vi "Stop Core.vi"(10 "final error code":i32, 11 "Debug UI in":refnum<class "Debug UI.lvclass">) -> (3 "Debug UI out":refnum<class "Debug UI.lvclass">)   [LabVIEW 2018, in "Assert API Components.lvlib" / "Log Assert Core.lvlib" / "Debug UI.lvclass"]
doc: "(<B>Filename</B>: Actor Framework.lvlib:Actor.lvclass:Stop Core.vi)\n\nDefines what the actor does before it stops. Use the <B>final error code</B> input to determine whether the actor shut down in response to an error.\n\nBy default, this method does nothing. A descendant class may override it to define behavior, such as shutting down any processes the actor initiated in its override of the Actor Core method."
uses:
  Debug UI.lvclass
  Debug UI.lvclass/Debug UI.ctl
  LAC Error Logger/LAC Error Logger.lvclass
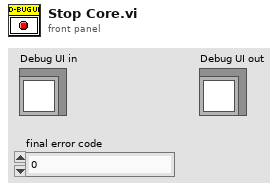
[diagram p1: front panel]
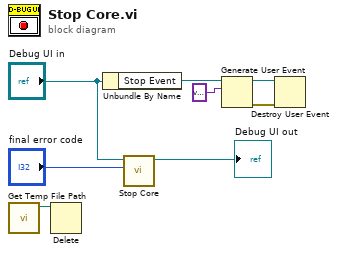
[diagram p0: block diagram]
diagram:
  n1 = call "Get Temp File Path.vi"() -> ("Temp File Path"=w1:path)  [unwired: 11 in]
  n2 = Delete(path (use dialog)=w1) -> ()  [unwired: 4 in, 3 out]
  n3 = Unbundle By Name("Debug UI in") -> ("Stop Event"=w5:refnum<user-event>)
  n4 = call-parent "Stop Core.vi"("final error code"="final error code", "Actor in"="Debug UI in") -> ("Actor out"=→"Debug UI out":refnum<class "Debug UI.lvclass">)  [unwired: 9 in]
  n5 = Generate User Event(user event=w5, event data cluster=variant ("event data")) -> (user event out=w3:refnum<user-event>, error out=w2:errorcluster)  [unwired: 2 in]
  n6 = Destroy User Event(user event=w3, error in=w2) -> ()  [unwired: 1 out]
